vi "Get Info.vi"(0 "Data in":refnum<class "Data.lvclass">, 5 "error in (no error)":errorcluster) -> (14 "Data out":refnum<class "Data.lvclass">, 15 "Class type out":u8, 16 "Data type out":u8, 17 "Data length out":i16, 18 "Dimensions out":i32[](array[numeric]), 19 "error out":errorcluster)   [LabVIEW 2012, in "MDSplus.lvlib" / "Data.lvclass"]
uses:
  <vilib>/MDSplus/Classes/Data_Class/Data.lvclass
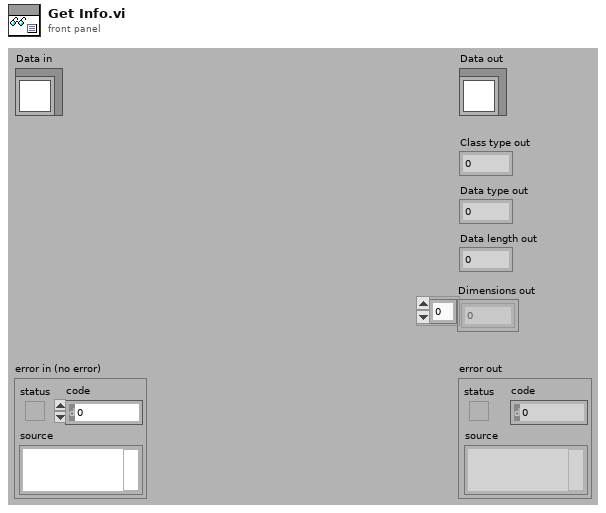
[diagram p1: front panel]
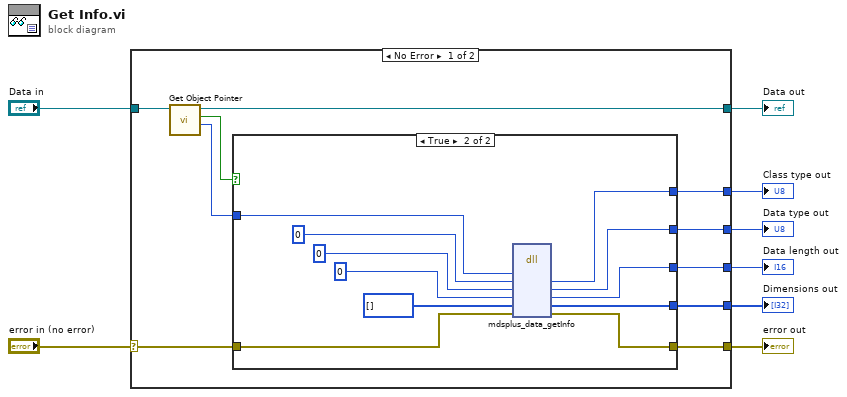
[diagram p0: block diagram]
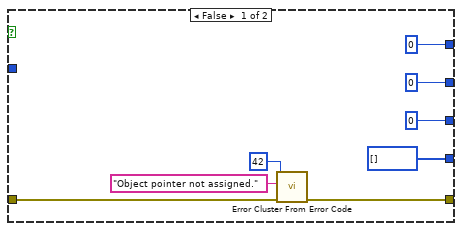
[diagram p2: hidden frame]
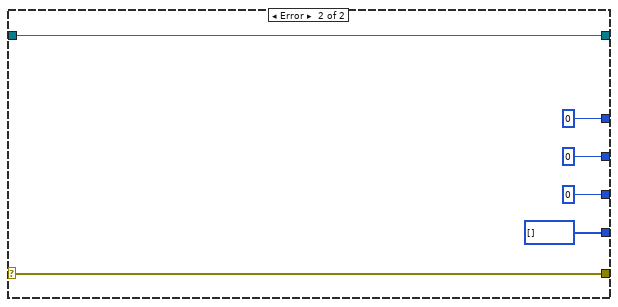
[diagram p3: hidden frame]
diagram:
  n1 = case shown="No Error" "error in (no error)" {
    selector: "error in (no error)" -> [w12 w43]
    tunnel: [w18 w43] -> w7
    tunnel: [w9 w42] -> w5
    tunnel: "Data in" -> [w17 w42]
    tunnel: [w16 u8 0 ("clazzOut")] -> w4
    tunnel: [w15 u8 0 ("dtypeOut")] -> w3
    tunnel: [w14 i16 0 ("lengthOut")] -> w2
    tunnel: [w13 i32[] [] ("lvIntArrHdlOut")] -> w1
    frame No Error {
      n2 = call-dynamic "Get Object Pointer.vi"("Data in"=w17) -> ("Object Pointer"=w10:i64, "Assigned object pointer?"=w11:bool, "Data out"=w9:refnum<class "Data.lvclass">)  [unwired: 8 in]
      n3 = case shown="True" w11 {
        tunnel: [w23 w37] -> w18
        tunnel: [u8 0 ("clazzOut") w32] -> w16
        tunnel: [u8 0 ("dtypeOut") w31] -> w15
        tunnel: [i16 0 ("lengthOut") w30] -> w14
        tunnel: [i32[] [] ("lvIntArrHdlOut") w29] -> w13
        tunnel: w12 -> [w24 w28]
        tunnel: w10 -> [_ w27]
        frame False {
          n4 = call <vilib>:"Error Cluster From Error Code.vi"("error in (no error)"=w24, "error message (\"\")"="Object pointer not assigned." ("error message (\"\")"), "error code (0)"=42) -> ("error out"=w23:errorcluster)  [unwired: 6 in]
        }
        frame True {
          n5 = dll-call lib="MDSobjectsLVShr" fn="mdsplus_data_getInfo"("lvDataPtr"=w27, "clazzOut"=u8 0, "dtypeOut"=u8 0, "lengthOut"=i16 0, "lvIntArrHdlOut"=i32[] [], "error"=w28) -> ("clazzOut"=w32:u8, "dtypeOut"=w31:u8, "lengthOut"=w30:i16, "lvIntArrHdlOut"=w29:i32[], "error"=w37:errorcluster)  [unwired: 5 in, 2 out]
        }
      }
    }
    frame Error {
    }
  }
  "error out" <- w7
  "Data out" <- w5
  "Class type out" <- w4
  "Data type out" <- w3
  "Data length out" <- w2
  "Dimensions out" <- w1
